vi "Run.vi"(7 "Team Index":i32, 8 "Column":i32, 9 "Row":i32, 10 "View":i32[](array[numeric]) caption="View (Team Index, -1: empty)", 11 "Defenders In":refnum<class "Defenders.lvclass">) -> (0 "Replicated":refnum<class "Square.lvclass">, 1 "Direction":T1, 2 "Action":T2, 3 "Square Out":refnum<class "Square.lvclass">)   [LabVIEW 2016, in "Defenders.lvclass"]
uses:
  Defenders.lvclass
  C:/Users/crwec/Desktop/Workspace/SquareBattle/Square/Square.lvclass
  Square/Square.lvclass
  Type Defs/Action Enum.ctl
  Type Defs/Direction Enum.ctl
  Common/Position.ctl
  Defenders.lvclass/Defenders.ctl
  SubVIs/Read-Only Globals.vi
  SubVIs/Globals (private).vi
  Common/Common.lvlib
  Type Defs/SB Type Defs.lvlib
panel:
  # "NW\nN\nNE\nE\nSE\nS\nSW\nW"
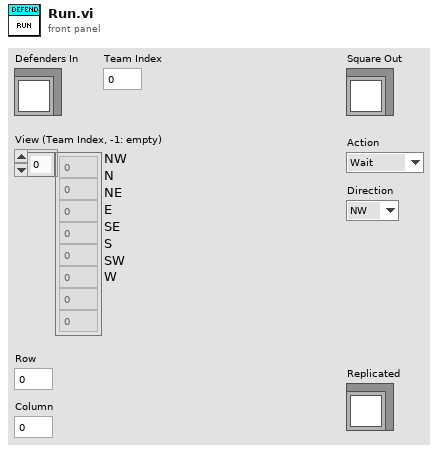
[diagram p1: front panel]
types:
  T1 = typedef "SB Type Defs.lvlib/Direction Enum.ctl" = enum16{"NW", "N", "NE", "E", "SE", "S", "SW", "W"}
  T2 = typedef "SB Type Defs.lvlib/Action Enum.ctl" = enum16{"Wait", "Move", "Attack", "Replicate"}
  T3 = typedef "Common.lvlib/Position.ctl" = cluster{"Column":i32, "Row":i32}
  T4 = typedef "Common.lvlib/Map DVR.ctl" = refnum<data-value>
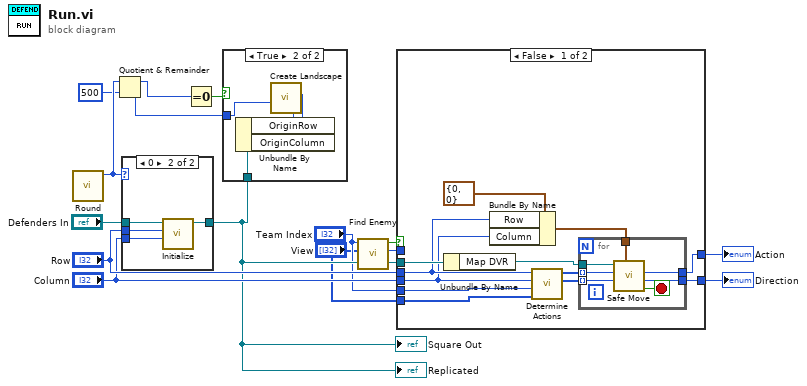
[diagram p0: block diagram]
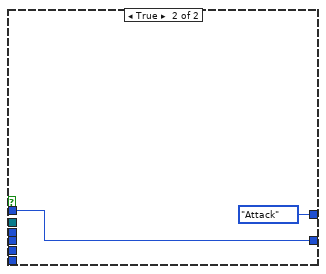
[diagram p3: hidden frame]
diagram:
  n1 = call "Round.vi"() -> ("Round"=w8:i32)  [unwired: 11 in]
  n2 = Quotient & Remainder(x=w8, y=500) -> (x-y*floor(x/y)=w5:i32, floor(x/y)=w4:i32)
  n3 = case shown="0" w8 {
    tunnel: "Defenders In" -> [w16 w20]
    tunnel: [w16 w19] -> w3
    tunnel: "Row" -> [_ w18]
    tunnel: "Column" -> [_ w17]
    frame Default {
    }
    frame 0 {
      n4 = call "Initialize.vi"("Column"=w17, "Row"=w18, "Defenders in"=w20) -> ("Defenders out"=w19:refnum<class "Defenders.lvclass">)  [unwired: 8 in]
    }
  }
  "Square Out" <- w3
  "Replicated" <- w3
  n5 = Equal To 0?(x=w5) -> (x = 0?=w6:bool)
  n6 = case shown="True" w6 {
    tunnel: w4 -> [_ w24]
    tunnel: w3 -> [_ w23]
    frame False {
    }
    frame True {
      n7 = Unbundle By Name(w23) -> ("OriginRow"=w22:i32, "OriginColumn"=w21:i32)
      n8 = call "Create Landscape.vi"("offset"=w24, "Column"=w21, "Row"=w22) -> ()  [unwired: 9 in]
    }
  }
  n9 = call "Find Enemy.vi"("View"="View", "Team Index"="Team Index") -> ("Direction"=w9:T1, "Found Enemy?"=w10:bool)  [unwired: 7 in, 1 out]
  n10 = case shown="False" w10 {
    tunnel: w3 -> [w36 _]
    tunnel: "Row" -> [w32 _]
    tunnel: "Column" -> [w31 _]
    tunnel: [w28 Action_Enum."Attack" ("Action")] -> w12
    tunnel: [w27 w45] -> w11
    tunnel: w9 -> [_ w45]
    tunnel: "Team Index" -> [w26 _]
    tunnel: "View" -> [w25 _]
    frame False {
      n11 = Unbundle By Name(w36) -> ("Map DVR"=w35:T4)
      n12 = Bundle By Name(cluster=T3 {"Column"=0, "Row"=0} ("Position in"), "Row"=w32, "Column"=w31) -> (w33:T3)
      n13 = call "Determine Actions.vi"("View"=w25, "Team Index"=w26, "Column"=w31, "Row"=w32) -> ("Directions"=w29:T1[], "Actions"=w30:T2[])  [unwired: 6 in]
      n14 = for {
        tunnel: w35 -> [w43]
        tunnel: w33 -> [w42]
        tunnel: w30 -> [w41] mode=indexing
        tunnel: w29 -> [w40] mode=indexing
        tunnel: [w38] -> w28
        tunnel: [w37] -> w27
        stop <- w39 stop-if-true
        n15 = call "Safe Move.vi"("Position in"=w42, "Direction in"=w40, "Desired Action"=w41, "Map DVR"=w43) -> ("Accepted?"=w39:bool, "Direction"=w37:T1, "Action"=w38:T2)  [unwired: 4 in, 1 out]
      }
    }
    frame True {
    }
  }
  "Action" <- w12
  "Direction" <- w11
